vi "断电保存变量.vi"() -> ()   [LabVIEW 2022 SP3, in "斯坦道多参数.lvlib"]
panel:
  in  "余氯":bool
  in  "悬浮物标液3":dbl
  in  "悬浮物标液2":dbl
  in  "悬浮物标液1":dbl
  in  "SS":bool
  in  "波特率":u32(ring)=115200 items=["115200"=115200, "9600"=9600]
  in  "水中油标液3":dbl
  in  "水中油标液2":dbl
  in  "水中油标液1":dbl
  in  "水中油":bool
  in  "氨氮标液3":dbl
  in  "COD标液3":dbl
  in  "氨氮标液2":dbl
  in  "氨氮标液1":dbl
  in  "COD标液2":dbl
  in  "COD标液1":dbl
  in  "氨氮":bool
  in  "氯化物标液3":dbl
  in  "氯化物标液2":dbl
  in  "氯化物标液1":dbl
  in  "氯化物":bool
  in  "Serial Config":T1={"baud rate (bps)"=9600, "stop bits"=10, "parity"=0, "flow control"=0, "timeout"=2000, "retries"=1} {"stop bits" items=["1.0"=10, "1.5"=15, "2.0"=20]; "parity" items=["None", "Odd", "Even", "Mark", "Space"]; "flow control" items=["None", "XON/XOFF", "RTS/CTS", "XON/XOFF & RTS/CTS", "DTR/DSR", "XON/XOFF & DTR/DSR"]}
  in  "藻密度单位":enum16{"cells/mL", "cells/L"}(ring)
  in  "叶绿素a单位":enum16{"μg/L", "mg/L"}(ring)
  in  "藻密度标液3":dbl
  in  "藻密度标液2":dbl
  in  "藻密度标液1":dbl
  in  "叶绿素a标液3":dbl
  in  "DO标液3":dbl=100.0
  in  "浊度标液3":dbl
  in  "orp标液3":dbl
  in  "电导率标液3":dbl
  in  "pH标液3":dbl
  in  "orp标液2":dbl
  in  "多机通讯":cluster{"开启":bool, "主站IP":string, "从站IP":string}={"开启"=FALSE, "主站IP"="192.168.1.100", "从站IP"="192.168.1.101"}
  in  "DO 2":bool
  in  "运行周期":T2
  in  "量程参数":T3={"水温 (℃)"={"量程下限"=0.0, "量程上限"=60.0}, "DO (mg/L)"={"量程下限"=0.0, "量程上限"=25.0}, "DO (%)"={"量程下限"=0.0, "量程上限"=250.0}, "pH"={"量程下限"=0.0, "量程上限"=14.0}, "电导率 (μS/cm)"={"量程下限"=0.0, "量程上限"=100000.0}, "盐度"={"量程下限"=0.0, "量程上限"=50.0}, "浊度 (NTU)"={"量程下限"=0.0, "量程上限"=1000.0}, "叶绿素a (μg/L)"={"量程下限"=0.0, "量程上限"=500.0}, "藻密度 (cells/mL)"={"量程下限"=0.0, "量程上限"=200000.0}, "ORP (mV)"={"量程下限"=-1999.0, "量程上限"=1999.0}, "氯化物（mg/L）"={"量程下限"=0.1, "量程上限"=20000.0}, "COD"={"量程下限"=0.0, "量程上限"=1000.0}, "氨氮"={"量程下限"=0.0, "量程上限"=1000.0}, "水中油"={"量程下限"=0.0, "量程上限"=1000.0}, "悬浮物"={"量程下限"=0.0, "量程上限"=1000.0}, "余氯"={"量程下限"=0.0, "量程上限"=5.0}}
  in  "COD":bool
  in  "水样测试组数":dbl=1.0 caption="水样测试组数:"
  in  "水样稳定时间":dbl=5.0 caption="水样稳定时间:"
  in  "滤波设置":T4={"pH"=2, "DO"=2, "Cond"=2, "Turb"=2, "叶绿素a"=2, "藻密度"=2, "ORP"=2, "COD"=2, "氯化物"=2, "氨氮"=2, "水中油"=2, "悬浮物"=2, "余氯"=2}
  in  "orp":bool
  in  "orp标液1":dbl
  in  "电导率标液2":dbl
  in  "电导率标液1":dbl
  in  "pH标液2":dbl
  in  "pH标液1":dbl
  in  "自动断线重连":bool=TRUE
  in  "藻密度":bool
  in  "连接方式":u16(ring) items=["Modbus RTU", "Modbus TCP"]
  in  "IP":string="192.168.1.206" caption="IP:"
  in  "Port":u16=502 caption="Port:"
  in  "定时控制输入":T5
  in  "探头选择":T7={"pH探头选择"=enum."STD", "DO探头选择"=enum."STD", "电导率探头选择"=enum."STD", "浊度探头选择"=enum."STD", "悬浮物探头选择"=enum."STD", "叶绿素a探头选择"=enum."STD", "蓝绿藻探头选择"=enum."纳清", "orp探头选择"=enum."国弘", "COD探头选择"=enum."国弘", "DO2探头选择"=enum."禹山", "氨氮探头选择"=enum."纳清", "水中油探头选择"=enum."国弘", "余氯探头选择"=enum."纳清"}
  in  "蓝绿藻":bool
  in  "盐度自动获取":bool=TRUE
  out "大气压补偿":dbl=101.35
  out "盐度补偿":dbl
  in  "浊度标液2":dbl
  in  "浊度标液1":dbl
  in  "DO标液2":dbl=100.0
  in  "DO标液1":dbl
  in  "叶绿素a标液2":dbl
  in  "叶绿素a标液1":dbl
  in  "叶绿素a启用":bool
  in  "标样核查配置":T8={"数据保存间隔"=1.0, "保存组数"=5.0, "水温标样值"=0.0, "pH标样值"=0.0, "溶解氧标样值"=0.0, "电导率标样值"=0.0, "浊度标样值"=0.0, "悬浮物标样值"=0.0, "叶绿素a标样值"=0.0, "藻密度标样值"=0.0, "ORP标样值"=0.0, "氯化物标样值"=0.0, "COD标样值"=0.0, "氨氮标样值"=0.0, "水中油标样值"=0.0, "余氯标样值"=0.0, "pH启用"=FALSE, "溶解氧启用"=FALSE, "电导率启用"=FALSE, "浊度启用"=FALSE, "悬浮物启用"=FALSE, "叶绿素a启用"=FALSE, "藻密度启用"=FALSE, "ORP启用"=FALSE, "氯化物启用"=FALSE, "COD启用"=FALSE, "氨氮启用"=FALSE, "水中油启用"=FALSE, "余氯启用"=FALSE}
  in  "Temp":bool=TRUE
  in  "Cond":bool=TRUE
  in  "Turb":bool=TRUE
  in  "DO":bool=TRUE
  in  "pH":bool=TRUE
  in  "VISA资源名称":refnum<visa-resource-name>="COM6"
  in  "水温通道":enum16{"pH", "DO", "浊度", "电导率", "叶绿素a", "藻密度"}(ring)
  # "请设置串口参数"
  # "请选择要启用的参数"
  # "运行模式："
  # "组"
  # "min"
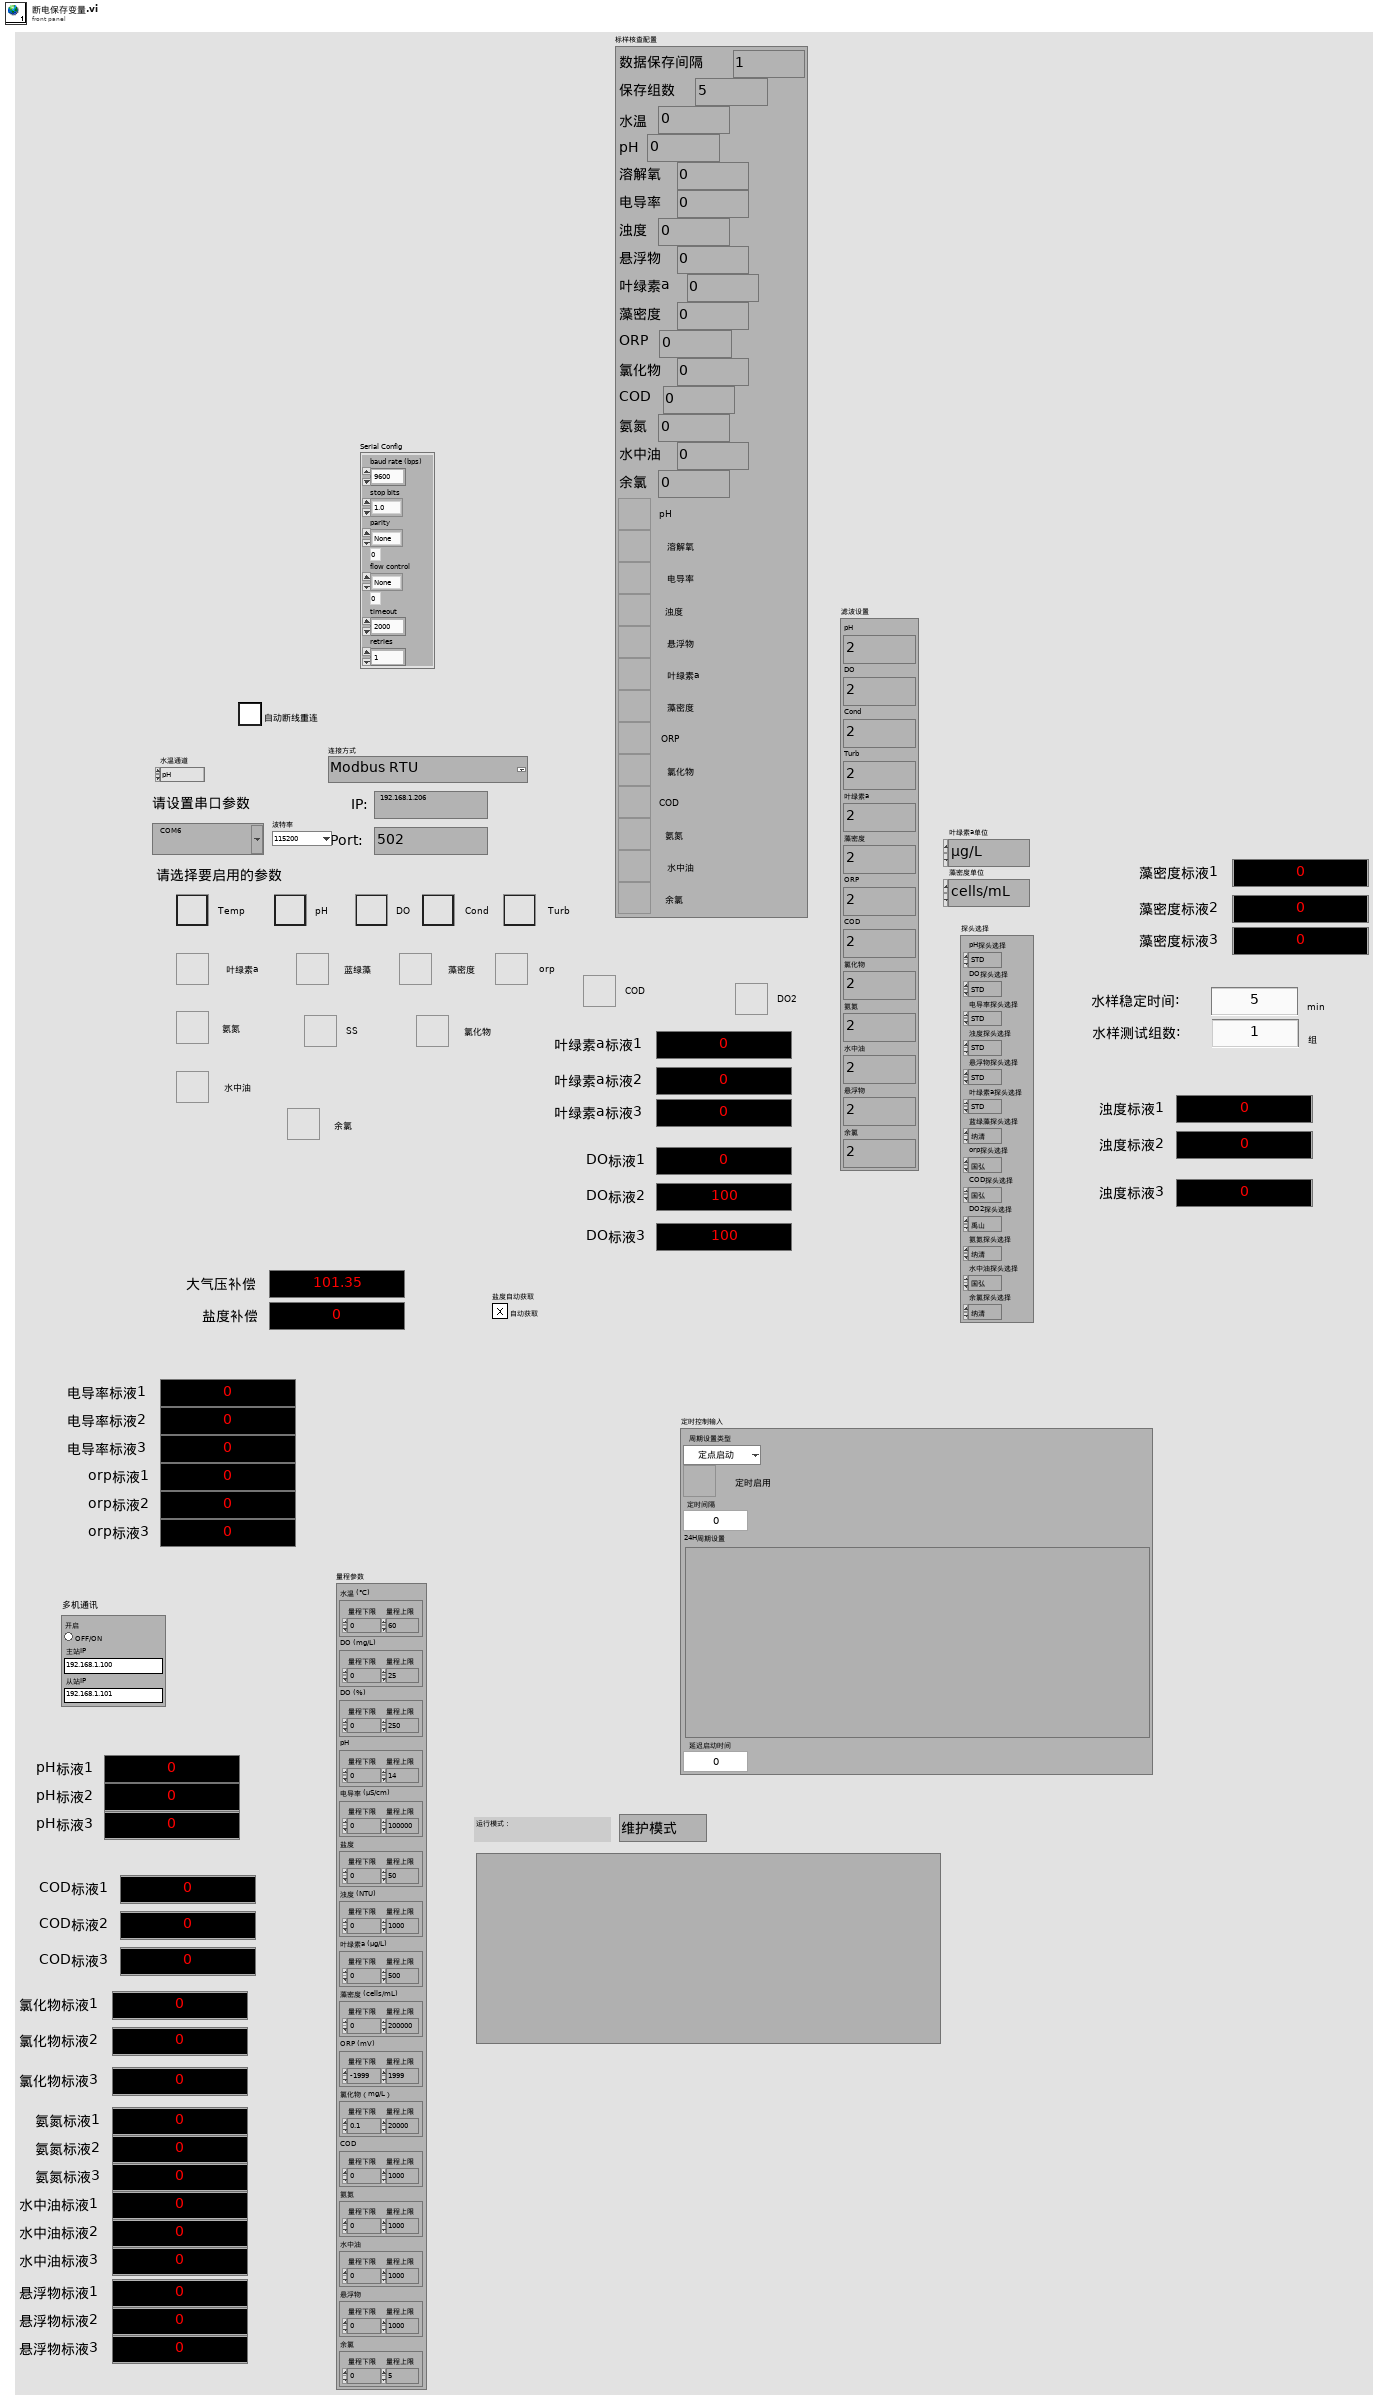
[diagram p1: front panel]
types:
  T1 = cluster{"baud rate (bps)":u32, "stop bits":u16, "parity":u16, "flow control":u16, "timeout":u32, "retries":i32}
  T2 = cluster{"运行模式":enum16{"维护模式", "常规模式", "应急模式", "质控模式"}, "24H周期设置":bool[]}
  T3 = cluster{"水温 (℃)":cluster{"量程下限":dbl, "量程上限":dbl}, "DO (mg/L)":cluster{"量程下限":dbl, "量程上限":dbl}, "DO (%)":cluster{"量程下限":dbl, "量程上限":dbl}, "pH":cluster{"量程下限":dbl, "量程上限":dbl}, "电导率 (μS/cm)":cluster{"量程下限":dbl, "量程上限":dbl}, "盐度":cluster{"量程下限":dbl, "量程上限":dbl}, "浊度 (NTU)":cluster{"量程下限":dbl, "量程上限":dbl}, "叶绿素a (μg/L)":cluster{"量程下限":dbl, "量程上限":dbl}, "藻密度 (cells/mL)":cluster{"量程下限":dbl, "量程上限":dbl}, "ORP (mV)":cluster{"量程下限":dbl, "量程上限":dbl}, "氯化物（mg/L）":cluster{"量程下限":dbl, "量程上限":dbl}, "COD":cluster{"量程下限":dbl, "量程上限":dbl}, "氨氮":cluster{"量程下限":dbl, "量程上限":dbl}, "水中油":cluster{"量程下限":dbl, "量程上限":dbl}, "悬浮物":cluster{"量程下限":dbl, "量程上限":dbl}, "余氯":cluster{"量程下限":dbl, "量程上限":dbl}}
  T4 = cluster{"pH":u32, "DO":u32, "Cond":u32, "Turb":u32, "叶绿素a":u32, "藻密度":u32, "ORP":u32, "COD":u32, "氯化物":u32, "氨氮":u32, "水中油":u32, "悬浮物":u32, "余氯":u32}
  T5 = cluster{"周期设置类型":enum16{"定点启动", "间隔启动"}, "定时功能启用":bool, "定时间隔":u32, "24H周期设置":bool[], "延迟启动时间":u32}
  T6 = typedef "斯坦道多参数.lvlib/探头类型.ctl" = enum16{"禹山", "国弘", "纳清", "STD"}
  T7 = cluster{"pH探头选择":T6, "DO探头选择":T6, "电导率探头选择":T6, "浊度探头选择":T6, "悬浮物探头选择":T6, "叶绿素a探头选择":T6, "蓝绿藻探头选择":T6, "orp探头选择":T6, "COD探头选择":T6, "DO2探头选择":T6, "氨氮探头选择":T6, "水中油探头选择":T6, "余氯探头选择":T6}
  T8 = cluster{"数据保存间隔":dbl, "保存组数":dbl, "水温标样值":dbl, "pH标样值":dbl, "溶解氧标样值":dbl, "电导率标样值":dbl, "浊度标样值":dbl, "悬浮物标样值":dbl, "叶绿素a标样值":dbl, "藻密度标样值":dbl, "ORP标样值":dbl, "氯化物标样值":dbl, "COD标样值":dbl, "氨氮标样值":dbl, "水中油标样值":dbl, "余氯标样值":dbl, "pH启用":bool, "溶解氧启用":bool, "电导率启用":bool, "浊度启用":bool, "悬浮物启用":bool, "叶绿素a启用":bool, "藻密度启用":bool, "ORP启用":bool, "氯化物启用":bool, "COD启用":bool, "氨氮启用":bool, "水中油启用":bool, "余氯启用":bool}
diagram:
